vi "CLSUIP_IsFpgaContext.vi"(0 "context":refnum<vi>, 11 "error in (no error)":errorcluster) -> (4 "context dup":refnum<vi>, 8 "is FPGA context":bool, 15 "error out":errorcluster)   [LabVIEW 2021, in "MemberVICreation.lvlib"]
uses:
  <resource>/Framework/Providers/LVClassLibrary/NewAccessors/MemberVICreation.lvlib
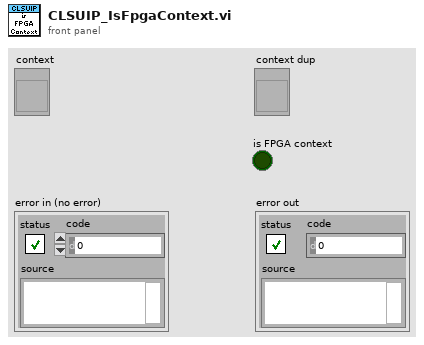
[diagram p1: front panel]
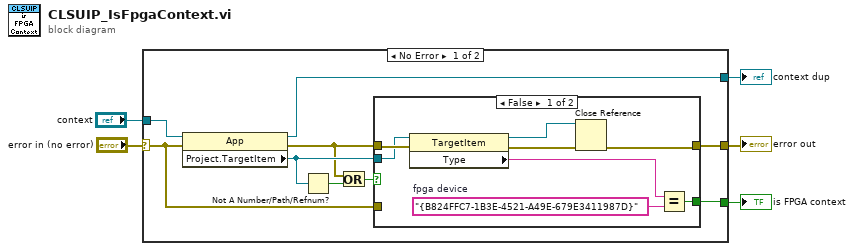
[diagram p0: block diagram]
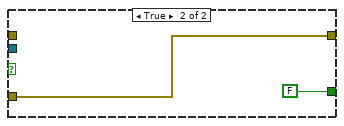
[diagram p2: hidden frame]
diagram:
  n1 = case shown="No Error" "error in (no error)" {
    selector: "error in (no error)" -> [w9 w26]
    tunnel: [w13 w26] -> w4
    tunnel: [w14 _] -> w3
    tunnel: "context" -> [w12 w25]
    tunnel: [w10 w25] -> w1
    frame No Error {
      n2 = property class="App"(reference=w12, error in=w9) -> (reference out=w10:refnum<vi>, error out=w7:errorcluster, "Project.TargetItem"=w11:refnum<vi>)
      n3 = Not A Number/Path/Refnum?(number/path/refnum=w11) -> (NaN/Path/Refnum?=w8:bool)
      n4 = Or(x=w7, y=w8) -> (x .or. y?=w6:bool)
      n5 = case shown="False" w6 {
        tunnel: w7 -> [w22 _]
        tunnel: [w19 FALSE] -> w14
        tunnel: [w15 w23] -> w13
        tunnel: w11 -> [w18 _]
        tunnel: w9 -> [_ w23]
        frame False {
          w21 = "{B824FFC7-1B3E-4521-A49E-679E3411987D}"  # fpga device
          n6 = property class="TargetItem"(reference=w18, error in=w22) -> (reference out=w16:refnum<vi>, error out=w17:errorcluster, "Type"=w20:string)
          n7 = Close Reference(reference=w16, error in (no error)=w17) -> (error out=w15:errorcluster)
          n8 = Equal?(x=w20, y=w21) -> (x = y?=w19:bool)
        }
        frame True {
        }
      }
    }
    frame Error {
    }
  }
  "error out" <- w4
  "is FPGA context" <- w3
  "context dup" <- w1
